vi "Read PumpState.vi"(11 "Pump_1AI_1DO_2DI in":refnum<class "PM_Group.lvclass">) -> (2 "PumpState":T1)   [LabVIEW 2019, in "PM_Group.lvclass"]
uses:
  PM_Group.lvclass
  TypeDef/StatePump.ctl
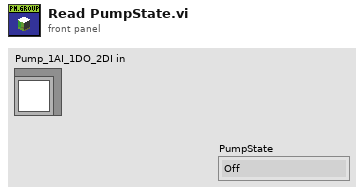
[diagram p1: front panel]
types:
  T1 = typedef "StatePump.ctl" = enum16{"Off", "TupningOn", "On", "TurningOff"}
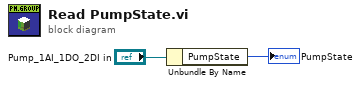
[diagram p0: block diagram]
diagram:
  n1 = Unbundle By Name("Pump_1AI_1DO_2DI in") -> ("PumpState"=→"PumpState":T1)
